vi "参数选择.vi"(11 "项名":string[](array[string])) -> (3 "字符串":string)   [LabVIEW 2016, in "下拉列表.xctl"]
uses:
  <vilib>/Utility/miscctls.llb/LVPointTypeDef.ctl
panel:
  in  "列表框":i32(listbox)
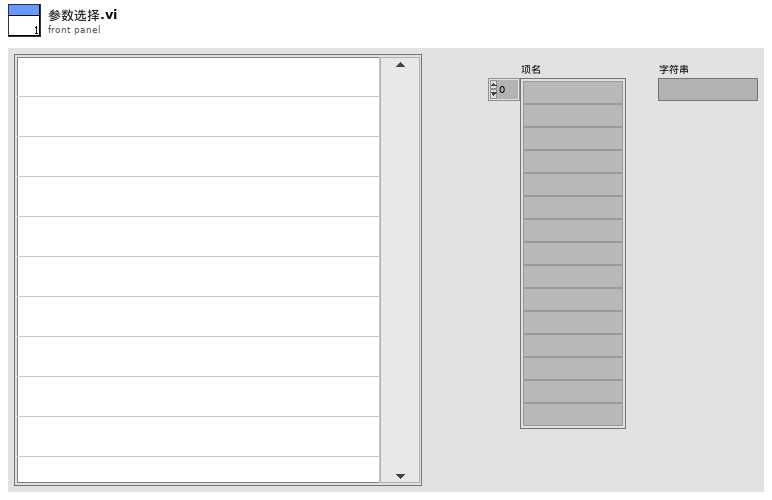
[diagram p1: front panel]
types:
  T1 = typedef "LVPointTypeDef.ctl" = cluster{"Horizontal":i16, "Vertical":i16}
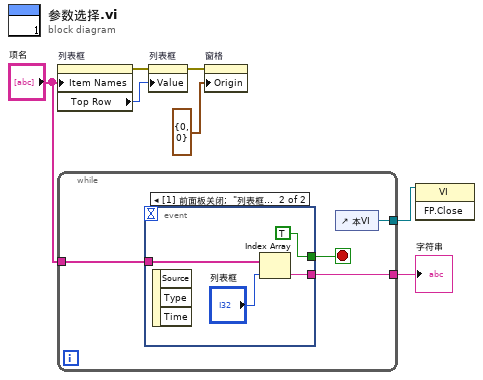
[diagram p0: block diagram]
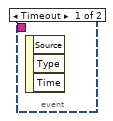
[diagram p2: hidden frame]
diagram:
  n1 = property on="列表框" class="LstBox (严格)"("Item Names"="项名") -> (error out=w2:errorcluster, "Top Row"=w3:i32)  [unwired: 2 in, 1 out]
  n2 = while {
    tunnel: "项名" -> [w11]
    tunnel: [w10] -> w7
    tunnel: [w8] -> w6
    stop <- w9 stop-if-true
    n3 = event shown="[1] 前面板关闭;  \"列表框\": 双击" {
      selector: _ -> [_ _]
      dyn-events: _ -> [_ _]
      timeout: _ -> [_ _]
      tunnel: w11 -> [_ w15]
      tunnel: [_ w13] -> w10
      tunnel: [_ TRUE] -> w9
      event Timeout {
        n4 = event-data() -> ()  [unwired: 1 in, 3 out]
      }
      event Panel Close; "列表框": Double Click {
        n5 = event-data() -> ()  [unwired: 1 in, 3 out]
        n6 = Index Array(array=w15, index="列表框") -> (element=w13:string)
      }
    }
    n7 = control-ref of="本VI"() -> (w8:refnum<vi>)
  }
  "字符串" <- w7
  n8 = property on="列表框" class="LstBox (严格)"(error in=w2, "Value"=w3) -> (error out=w1:errorcluster)  [unwired: 1 in, 1 out]
  n9 = property on="窗格" class="Pane"(error in=w1, "Origin"=T1 {"Horizontal"=0, "Vertical"=0} ("原点")) -> ()  [unwired: 1 in, 2 out]
  n10 = invoke class="VI" method="FP.Close"(reference=w6) -> ()  [unwired: 2 in, 3 out]
